vi "Append Front Panel Image to Report (path) shell.vi"(4 "Image Format (jpeg)":enum32{"PNG", "JPEG", "GIF"}(ring)=enum."JPEG", 5 "visible area only?":bool, 6 "alignment (default)":T1, 7 "error in (no error)":errorcluster, 8 "description":string, 9 "VI":path, 10 "report in":T2) -> (0 "error out":errorcluster, 2 "VI path out":path, 3 "report out":T2)   [LabVIEW 2017]
doc: "Creates an image of the front panel of the VI you specify in <B>VI</B> and appends it to a report. The data type you wire to the <B>VI</B> input determines the polymorphic instance to use."
uses:
  <vilib>/Utility/NIReport.llb/Generate Report Object Reference.ctl
  <vilib>/Utility/NIReport.llb/NI_report.lvclass
  <vilib>/Utility/NIReport.llb/HTML Report Image Alignment.ctl
  <vilib>/Utility/NIReport.llb/NI_ReportGenerationCore.lvlib
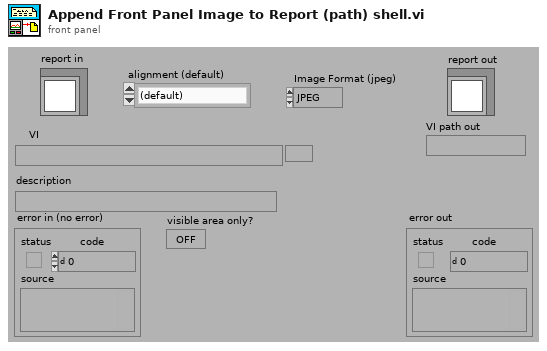
[diagram p1: front panel]
types:
  T1 = typedef "NI_ReportGenerationCore.lvlib/HTML Report Image Alignment.ctl" = enum16{"(default)", "LEFT", "RIGHT", "TOP", "TEXTTOP", "MIDDLE", "ABSMIDDLE", "BASELINE", "BOTTOM", "ABSBOTTOM"}
  T2 = typedef "Generate Report Object Reference.ctl" = refnum<class "NI_report.lvclass">
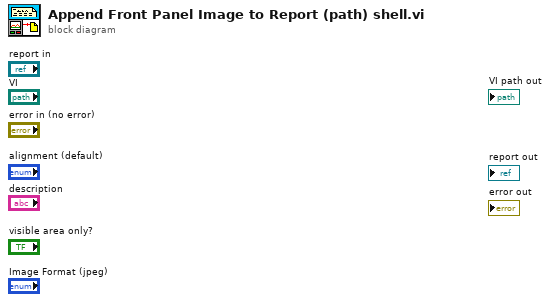
[diagram p0: block diagram]
diagram:
